vi "Actor Create.vi"(9 "Nested Alias":string, 10 "Nested Actor":refnum<class "Actor.lvclass">, 11 "Actor Create in":refnum<class "Actor Create.lvclass">) -> (3 "Actor Create out":refnum<class "Actor Create.lvclass">)   [LabVIEW 2021, in "Actor Create.lvlib" / "Actor Create.lvclass"]
uses:
  Actor Create.lvclass
  jettl/Actor/Actor.lvclass
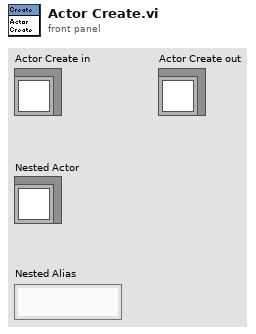
[diagram p1: front panel]
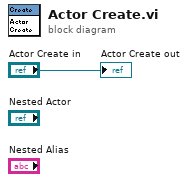
[diagram p0: block diagram]
diagram:
  "Actor Create out" <- "Actor Create in"
